vi "Empty Host Resources.vi"() -> (0 "Host Resources":T1)   [LabVIEW 2021, in "Acquisition.lvlib"]
doc: "(inline VI) Return an empty Host Resources. Use in-place of a block diagram constant.\n\nA cluster representing the resources on the running Host system: 1. an array of installed packages and 2. an array of discovered IO devices."
uses:
  Acquisition.lvlib
  Host Resources.ctl
  Host Software Package.ctl
  Host IO Resource.ctl
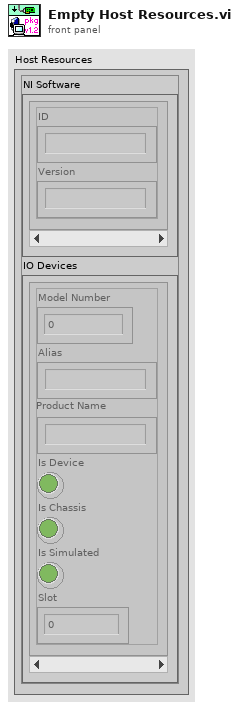
[diagram p1: front panel]
types:
  T1 = typedef "Acquisition.lvlib/Host Resources.ctl" = cluster{"NI Software":T2[], "IO Devices":T3[]}
  T2 = typedef "Acquisition.lvlib/Host Software Package.ctl" = cluster{"ID":string, "Version":string}
  T3 = typedef "Acquisition.lvlib/Host IO Resource.ctl" = cluster{"Model Number":u32, "Alias":string, "Product Name":string, "Is Device":bool, "Is Chassis":bool, "Is Simulated":bool, "Slot":i32}
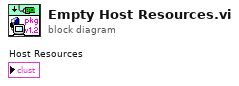
[diagram p0: block diagram]
diagram:
